vi "DummyVI.vi"(8 "error in":errorcluster, 11 "Monitor":u16) -> (0 "error out":errorcluster, 1 "Array":u16[](array[numeric]), 2 "Array 2":u16[](array[numeric]), 3 "FP:Window Size":cluster{"Width":i16, "Height":i16})   [LabVIEW 2014]
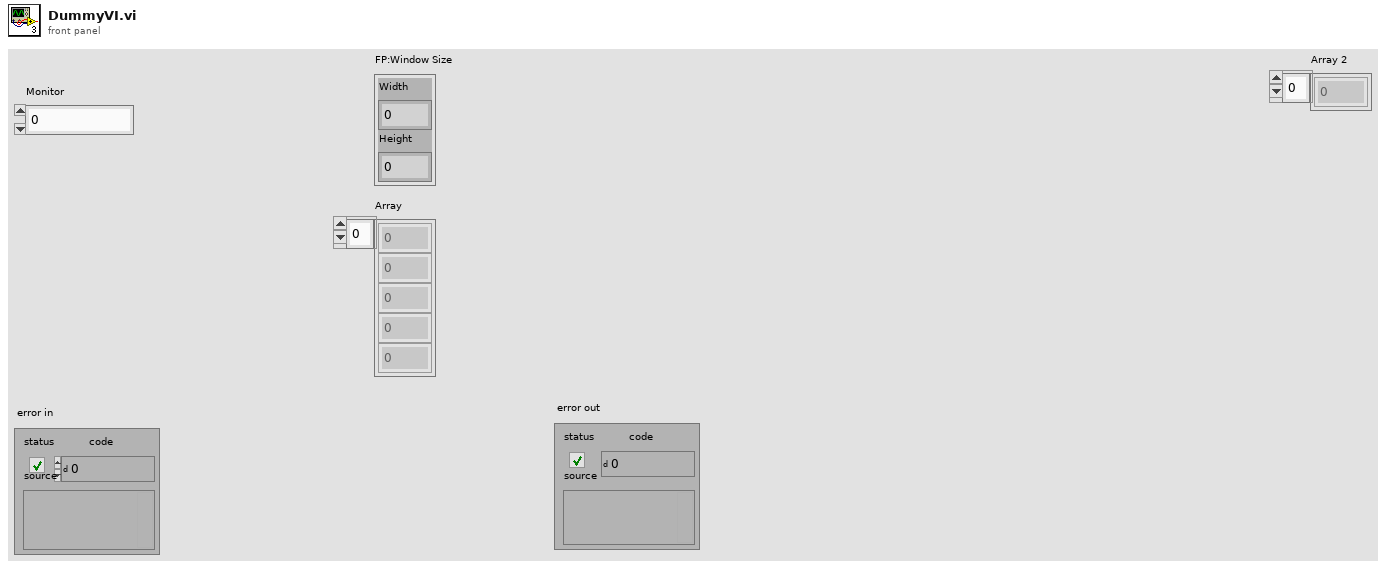
[diagram p1: front panel]
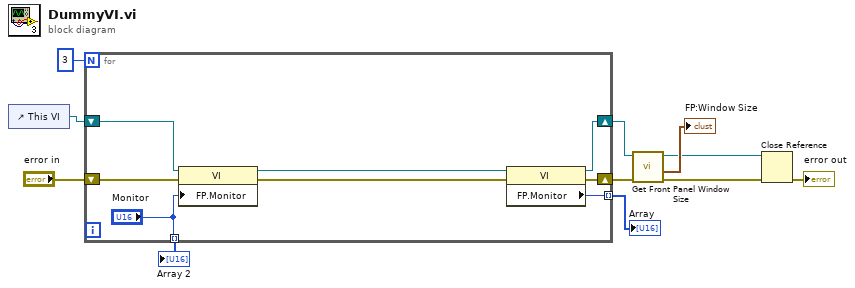
[diagram p0: block diagram]
diagram:
  n1 = control-ref of="This VI"() -> (w1:refnum<vi>)
  n2 = for {
    N: 3 -> [_]
    shift-right: [w15] -> w9
    shift-left: w1 -> [w19]
    shift-right: [w16] -> w10
    shift-left: "error in" -> [w18]
    tunnel: [w17] -> w5 mode=indexing
    tunnel: ["Monitor"] -> w2 mode=indexing
    n3 = property class="VI"(reference=w19, error in=w18, "FP.Monitor"="Monitor") -> (reference out=w13:refnum<vi>, error out=w14:errorcluster)
    n4 = property class="VI"(reference=w13, error in=w14) -> (reference out=w15:refnum<vi>, error out=w16:errorcluster, "FP.Monitor"=w17:u16)
  }
  "Array" <- w5
  "Array 2" <- w2
  n5 = call "Get Front Panel Window Size.vi"("error in"=w10, "VI Ref"=w9) -> ("error out"=w3:errorcluster, "FP:Window Size"=→"FP:Window Size":cluster{"Width":i16, "Height":i16}, "VI Ref"=w4:refnum<vi>)  [unwired: 4 in, 3 out]
  n6 = Close Reference(reference=w4, error in (no error)=w3) -> (error out=→"error out":errorcluster)
